vi "Scripting_FixBrokenVI.vi"(7 "AppRef":refnum<vi>, 8 "error in (no error)":errorcluster, 11 "ViPath/ViName":variant) -> (0 "error out":errorcluster)   [LabVIEW 2014, in "Scripting.lvclass"]
uses:
  <resource>/Framework/Providers/Open_GDS/ClassProviders/Common/ScriptingFunctions/Scripting.lvclass
  <vilib>/Utility/traverseref.llb/TRef TravTarget.ctl
  <vilib>/Utility/traverseref.llb/VI Scripting - Traverse.lvlib
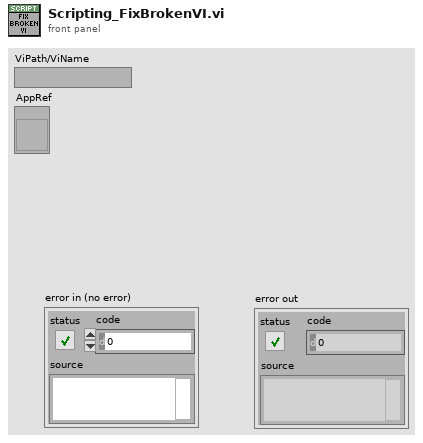
[diagram p1: front panel]
types:
  T1 = typedef "TRef TravTarget.ctl" = enum16{"FP", "BD", "Other"}
  T2 = enum32{"Bad", "Idle", "Run top level", "Running"}
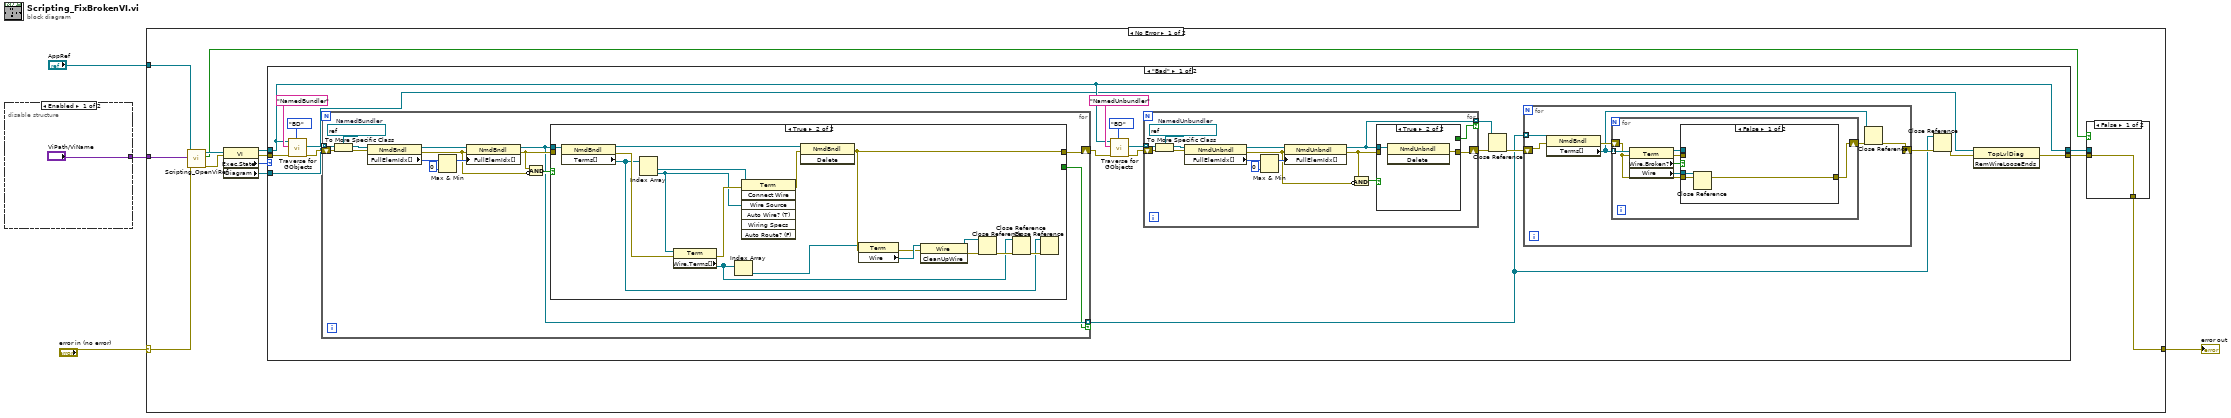
[diagram p0: block diagram]
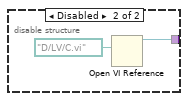
[diagram p2: hidden frame]
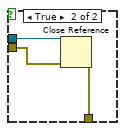
[diagram p3: hidden frame]
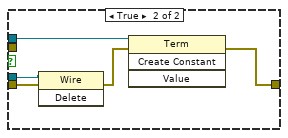
[diagram p4: hidden frame]
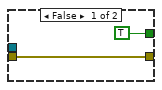
[diagram p5: hidden frame]
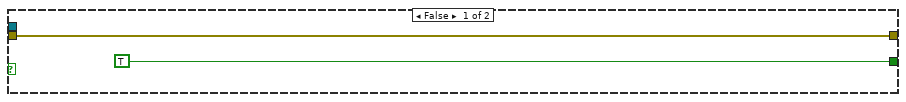
[diagram p6: hidden frame]
diagram:
  n1 = disable-structure shown="Enabled" {
    disable-tunnel: ["ViPath/ViName" w7] -> w4
    frame Enabled {
    }
    frame Disabled {
      n2 = Open VI Reference(vi path=path "D:/LV/C.vi") -> (vi reference=w7:refnum<vi>)  [unwired: 5 in, 1 out]
    }
  }
  n3 = case shown="No Error" "error in (no error)" {
    selector: "error in (no error)" -> [w18 w119]
    tunnel: w4 -> [w20 _]
    tunnel: "AppRef" -> [w19 _]
    tunnel: [w10 w119] -> w1
    frame No Error {
      n4 = call <resource>:"Scripting_OpenViRef.vi"("error in"=w18, "ViPath/ViName/Viref"=w20, "AppRef"=w19) -> ("error out"=w16:errorcluster, "RefOpened(Needs to be closed)"=w9:bool, "vi reference"=w17:refnum<vi>)  [unwired: 6 in]
      n5 = property class="VI"(reference=w17, error in=w16) -> (reference out=w14:refnum<vi>, error out=w12:errorcluster, "Exec.State"=w15:T2, "Diagram"=w8:refnum<vi>)
      n6 = case shown="\"Bad\"" w15 {
        tunnel: w14 -> [w34 w118]
        tunnel: [w34 w118] -> w13
        tunnel: w12 -> [w43 w117]
        tunnel: [w25 w117] -> w11
        tunnel: w8 -> [w27 _]
        frame "Bad" {
          n7 = call <vilib>:"Traverse for GObjects.vi"("Traverse Target"=TRef_TravTarget."BD", "error in (no error)"=w43, "Class Name"="NamedBundler", "VI Refnum"=w34) -> ("error out"=w39:errorcluster, "References"=w40:refnum<vi>[])  [unwired: 4 in, 2 out]
          n8 = for {
            tunnel: w40 -> [w97] mode=indexing
            shift-right: [w83] -> w35
            shift-left: w39 -> [w95]
            tunnel: [w85] -> w30 mode=indexing if=w84
            w96 = refnum<vi> refnum  # NamedBundler
            n9 = To More Specific Class(target class=w96, reference=w97, error in=w95) -> (specific class reference=w94:refnum<vi>, error out=w93:errorcluster)
            n10 = property class="NmdBndl"(reference=w94, error in=w93) -> (reference out=w92:refnum<vi>, error out=w88:errorcluster, "FullElemIdx[]"=w91:i32[])
            n11 = Max & Min(x=w91, y=0) -> (max(x,y)=w89:i32[])  [unwired: 1 out]
            n12 = property class="NmdBndl"(reference=w92, error in=w88, "FullElemIdx[]"=w89) -> (reference out=w85:refnum<vi>, error out=w86:errorcluster)
            n13 = Compound Arithmetic op=AND(w86, invert w88) -> (w87:bool)
            n14 = case shown="True" w87 {
              tunnel: w85 -> [_ w116]
              tunnel: w86 -> [w99 _]
              tunnel: [w99 w109] -> w83
              tunnel: [TRUE _] -> w84
              frame False {
              }
              frame True {
                n15 = property class="NmdBndl"(reference=w116) -> (reference out=w115:refnum<vi>, error out=w112:errorcluster, "Terms[]"=w101:refnum<vi>[])  [unwired: 1 in]
                n16 = Index Array(array=w101) -> (element #1=w100:refnum<vi>, element #2=w104:refnum<vi>)  [unwired: 2 in]
                n17 = property class="Term"(reference=w104, error in=w112) -> (error out=w111:errorcluster, "Wire.Terms[]"=w103:refnum<vi>[])  [unwired: 1 out]
                n18 = Index Array(array=w103) -> (element=w108:refnum<vi>)  [unwired: 1 in]
                n19 = invoke class="Term" method="Connect Wire"(reference=w100, error in=w111, "Wire Source"=w104) -> (error out=w110:errorcluster)  [unwired: 4 in, 6 out]
                n20 = invoke class="NmdBndl" method="Delete"(reference=w115, error in=w110) -> (error out=w109:errorcluster)  [unwired: 1 in, 2 out]
                n21 = property class="Term"(reference=w108, error in=w109) -> (error out=w106:errorcluster, "Wire"=w107:refnum<vi>)  [unwired: 1 out]
                n22 = invoke class="Wire" method="CleanUpWire"(reference=w107, error in=w106) -> (reference out=w113:refnum<vi>, error out=w114:errorcluster)  [unwired: 1 in, 1 out]
                n23 = Close Reference(reference=w113, error in (no error)=w114) -> (error out=w105:errorcluster)
                n24 = Close Reference(reference=w103, error in (no error)=w105) -> (error out=w102:errorcluster)
                n25 = Close Reference(reference=w101, error in (no error)=w102) -> ()  [unwired: 1 out]
              }
            }
          }
          n26 = call <vilib>:"Traverse for GObjects.vi"("Traverse Target"=TRef_TravTarget."BD", "error in (no error)"=w35, "Class Name"="NamedUnbundler", "VI Refnum"=w34) -> ("error out"=w38:errorcluster, "References"=w29:refnum<vi>[])  [unwired: 4 in, 2 out]
          n27 = for {
            tunnel: w29 -> [w78] mode=indexing
            shift-right: [w66] -> w33
            shift-left: w38 -> [w76]
            tunnel: [w65] -> w28 mode=indexing if=w64
            w77 = refnum<vi> refnum  # NamedUnbundler
            n28 = To More Specific Class(target class=w77, reference=w78, error in=w76) -> (specific class reference=w75:refnum<vi>, error out=w74:errorcluster)
            n29 = property class="NmdUnbndl"(reference=w75, error in=w74) -> (reference out=w73:refnum<vi>, error out=w69:errorcluster, "FullElemIdx[]"=w72:i32[])
            n30 = Max & Min(x=w72, y=0) -> (max(x,y)=w70:i32[])  [unwired: 1 out]
            n31 = property class="NmdUnbndl"(reference=w73, error in=w69, "FullElemIdx[]"=w70) -> (reference out=w65:refnum<vi>, error out=w67:errorcluster)
            n32 = Compound Arithmetic op=AND(w67, invert w69) -> (w68:bool)
            n33 = case shown="True" w68 {
              tunnel: w65 -> [_ w82]
              tunnel: w67 -> [w80 _]
              tunnel: [w80 w81] -> w66
              tunnel: [TRUE _] -> w64
              frame False {
              }
              frame True {
                n34 = invoke class="NmdUnbndl" method="Delete"(reference=w82) -> (error out=w81:errorcluster)  [unwired: 2 in, 2 out]
              }
            }
          }
          n35 = Close Reference(reference=w28, error in (no error)=w33) -> (error out=w32:errorcluster)
          n36 = for {
            shift-right: [w45] -> w31
            shift-left: w32 -> [w48]
            tunnel: w30 -> [w49] mode=indexing
            n37 = property class="NmdBndl"(reference=w49, error in=w48) -> (error out=w47:errorcluster, "Terms[]"=w44:refnum<vi>[])  [unwired: 1 out]
            n38 = for {
              tunnel: w44 -> [w56] mode=indexing
              shift-right: [w53] -> w46
              shift-left: w47 -> [w51]
              n39 = property class="Term"(reference=w56, error in=w51) -> (reference out=w52:refnum<vi>, error out=w50:errorcluster, "Wire.Broken?"=w54:bool, "Wire"=w55:refnum<vi>)
              n40 = case shown="False" w54 {
                tunnel: w55 -> [w57 w63]
                tunnel: w51 -> [w58 w62]
                tunnel: [w58 w59] -> w53
                tunnel: w52 -> [_ w61]
                tunnel: w50 -> [_ _]
                frame False {
                  n41 = Close Reference(reference=w57) -> ()  [unwired: 1 in, 1 out]
                }
                frame True {
                  n42 = invoke class="Wire" method="Delete"(reference=w63, error in=w62) -> (error out=w60:errorcluster)  [unwired: 1 in, 2 out]
                  n43 = invoke class="Term" method="Create Constant"(reference=w61, error in=w60) -> (error out=w59:errorcluster)  [unwired: 2 in, 3 out]
                }
              }
            }
            n44 = Close Reference(reference=w44, error in (no error)=w46) -> (error out=w45:errorcluster)
          }
          n45 = Close Reference(reference=w30, error in (no error)=w31) -> (error out=w26:errorcluster)
          n46 = invoke class="TopLvlDiag" method="RemWireLooseEnds"(reference=w27, error in=w26) -> (error out=w25:errorcluster)  [unwired: 1 in, 2 out]
        }
        frame "Idle", Default {
        }
      }
      n47 = case shown="False" w9 {
        tunnel: w13 -> [_ w24]
        tunnel: w11 -> [w21 w23]
        tunnel: [w21 w22] -> w10
        frame False {
        }
        frame True {
          n48 = Close Reference(reference=w24, error in (no error)=w23) -> (error out=w22:errorcluster)
        }
      }
    }
    frame Error {
    }
  }
  "error out" <- w1
